vi "parser-main.vi"() -> ()   [LabVIEW 2017, in "automode.lvlib"]
uses:
  automode.lvlib
panel:
  in  "Codes handled":string[](array[string])
  in  "Subsytem name":string
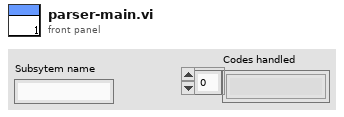
[diagram p1: front panel]
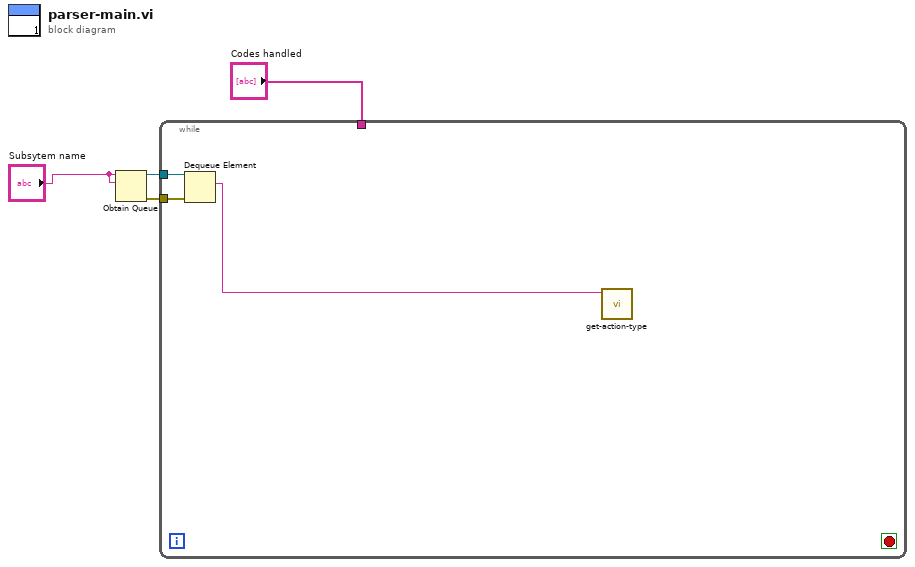
[diagram p0: block diagram]
diagram:
  n1 = Obtain Queue(name (unnamed)="Subsytem name", element data type="Subsytem name") -> (queue out=w2:refnum<queue>, error out=w3:errorcluster)  [unwired: 3 in, 1 out]
  n2 = while {
    tunnel: w3 -> [w7]
    tunnel: w2 -> [w6]
    tunnel: "Codes handled" -> [_]
    stop <- _ stop-if-true
    n3 = Dequeue Element(queue=w6, error in (no error)=w7) -> (element=w5:string)  [unwired: 1 in, 3 out]
    n4 = call "get-action-type.vi"("Subsytem name"=w5) -> ()  [unwired: 11 in]
  }
